vi "factorial.vi"(10 "n":u32) -> (2 "n!":u64)   [LabVIEW 2019]
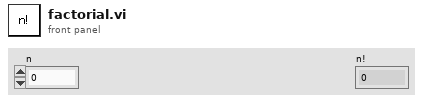
[diagram p1: front panel]
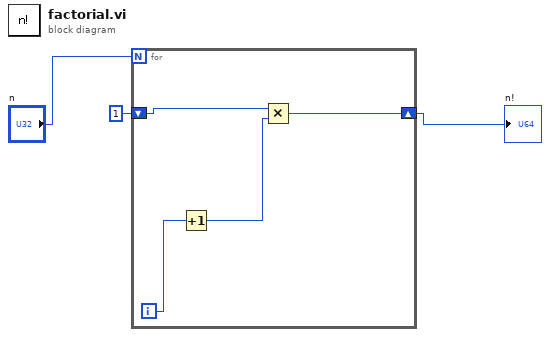
[diagram p0: block diagram]
diagram:
  n1 = for {
    N: "n" -> [_]
    shift-right: [w7] -> w1
    shift-left: 1 -> [w6]
    i -> [w5]
    n2 = Increment(x=w5) -> (x+1=w4:i32)
    n3 = Multiply(x=w6, y=w4) -> (x*y=w7:i32)
  }
  "n!" <- w1
